vi "PID Signal.vi"(1 "Tracking errors, e":dbl[](array[numeric]) format="%.3f", 2 "Gains, Ks":dbl[](array[numeric]) format="%.3f", 3 "Control, u(k)":dbl=1.0 min=-40.0 max=40.0 step=5.0 format="%.2f") -> (0 "Control, u(k+1)":dbl=1.0 min=-40.0 max=40.0 step=5.0 format="%.2f")   [LabVIEW 2022 SP3]
uses:
  <vilib>/express/express arith-compare/Formula/XNode/ExpressFormulaBlockNode.xnode
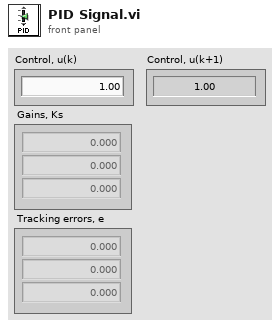
[diagram p1: front panel]
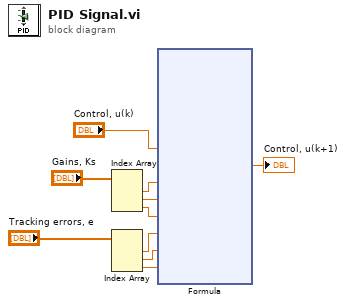
[diagram p0: block diagram]
diagram:
  n1 = Index Array(array="Gains, Ks") -> (element #1=w6:dbl, element #2=w5:dbl, element #3=w4:dbl)  [unwired: 3 in]
  n2 = Index Array(array="Tracking errors, e") -> (element #1=w3:dbl, element #2=w2:dbl, element #3=w1:dbl)  [unwired: 3 in]
  n3 = xnode "Formula"("u"="Control, u(k)", "kp"=w6, "ki"=w5, "kd"=w4, "e1"=w3, "e2"=w2, "e3"=w1) -> ("Result"=→"Control, u(k+1)":dbl)  [unwired: 1 in, 1 out]
